vi "Bot.vi"(7 "BotData":T4, 11 "GameState":T2) -> (0 "error out":errorcluster, 3 "Move":T1)   [LabVIEW 2015, in "ManualBot.lvlib"]
uses:
  ManualBot.lvlib
  TronVIEWBotAPI/MovementDirection.ctl
  TronVIEWBotAPI/BotData.ctl
  TronVIEWBotAPI/GameState.ctl
  TronviewGame/Board/Position.ctl
  TronVIEWBotAPI/TronVIEWBotAPI.lvlib
  TronviewGame/Board/Board.lvclass
panel:
  in  "Move 2":T1
  in  "Move":bool
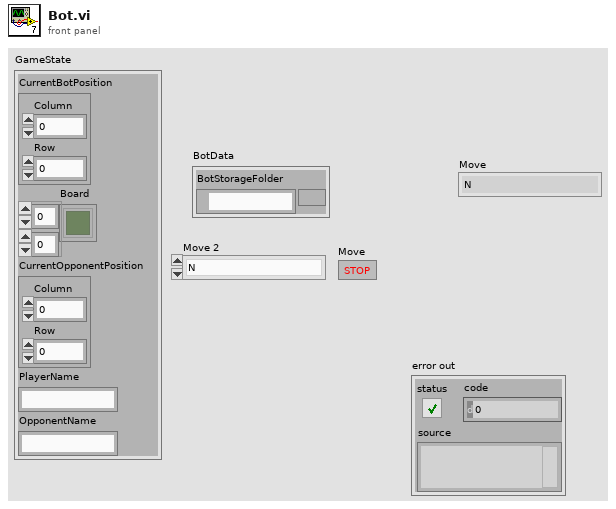
[diagram p1: front panel]
types:
  T1 = typedef "TronVIEWBotAPI.lvlib/MovementDirection.ctl" = enum16{"N", "S", "W", "E"}
  T2 = typedef "TronVIEWBotAPI.lvlib/GameState.ctl" = cluster{"CurrentBotPosition":T3, "Board":bool[][], "CurrentOpponentPosition":T3, "PlayerName":string, "OpponentName":string}
  T3 = typedef "TronviewGame.lvlib/Board.lvclass/Position.ctl" = cluster{"Column":i32, "Row":i32}
  T4 = typedef "TronVIEWBotAPI.lvlib/BotData.ctl" = cluster{"BotStorageFolder":path}
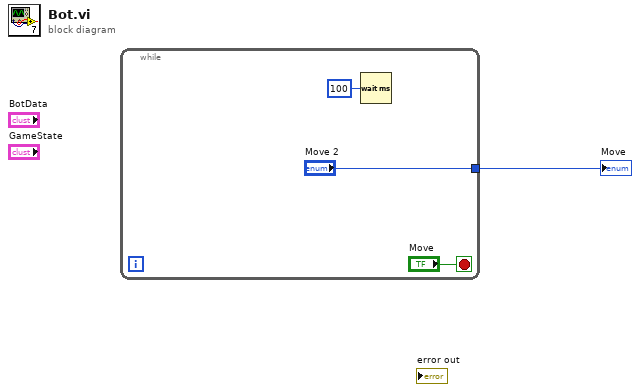
[diagram p0: block diagram]
diagram:
  n1 = while {
    tunnel: ["Move 2"] -> w1
    stop <- "Move" stop-if-true
    n2 = Wait (ms)(milliseconds to wait=u32 100) -> ()  [unwired: 1 out]
  }
  "Move" <- w1
